vi "PCO_SetCameraSetup.vi"(8 "error in (no error)":errorcluster {"code" format="%x"}, 9 "dwSetup":u32[](array[numeric]), 10 "wType":u16, 11 "ph":u64) -> (0 "error out":errorcluster {"code" format="%x"}, 2 "ErrorMessage":i32 format="%x", 3 "ph out":u64)   [LabVIEW 2019, in "SDK.lvlib" / "GeneralCameraControl.lvlib"]
doc: "<b>Description</b>\nCommand can be used to set the shutter mode of a pco.edge.This function is used to set the operation mode of the camera. If operation mode is changed, PCO_RebootCamera must be called afterwards. It is recommended to set the command timeout to 2000 ms by calling PCO_SetTimeouts before changing the setup.\n\n<b>Supported camera type:</b>\npco.edge\n\n<b>Descriptor dependency:</b>\nNone"
uses:
  GeneralCameraControl.lvlib
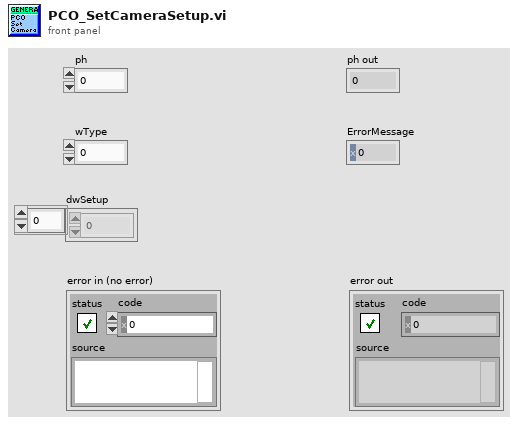
[diagram p1: front panel]
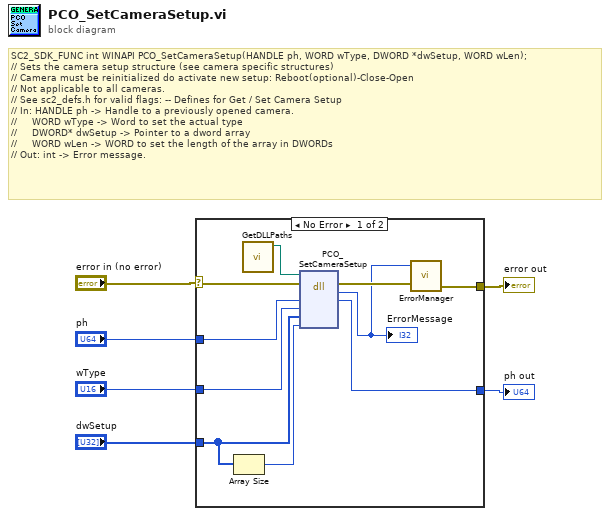
[diagram p0: block diagram]
diagram:
  # "SC2_SDK_FUNC int WINAPI PCO_SetCameraSetup(HANDLE ph, WORD wType, DWORD *dwSetup, WORD wLen);\n// Sets the camera setup structure (see camera specific structures)\n// Camera must be reinitialized do activate new setup: Reboot(optional)-Close-Open\n// Not applicable to all cameras.\n// See sc2_defs.h for valid flags: -- Defines for Get / Set Camera Setup\n// In: HANDLE ph -> Handle to a previously opened camera.\n//     WORD wType -> Word to set the actual type\n//     DWORD* dwSetup -> Pointer to a dword array\n//     WORD wLen -> WORD to set the length of the array in DWORDs\n// Out: int -> Error message."
  n1 = case shown="No Error" "error in (no error)" {
    selector: "error in (no error)" -> [w12 w18]
    tunnel: "ph" -> [w16 w17]
    tunnel: [w15 w17] -> w5
    tunnel: [w14 w18] -> w4
    tunnel: "dwSetup" -> [w9 _]
    tunnel: "wType" -> [w10 _]
    frame No Error {
      n2 = Array Size(array=w9) -> (size(s)=w8:i32)
      n3 = call "GetDLLPaths.vi"() -> ("SC2_Cam_Path"=w7:path)  [unwired: 9 in, 2 out]
      n4 = dll-call lib="?" fn="PCO_SetCameraSetup"(path in=w7, error in=w12, "ph"=w16, "wType"=w10, "dwSetup"=w9, "wLen"=w8) -> (error out=w13:errorcluster, "return type"=w11:i32, "ph"=w15:u64)  [unwired: 4 in, 1 out]
      "ErrorMessage" <- w11
      n5 = call "ErrorManager.vi"("error in (no error)"=w13, "error code"=w11) -> ("error out"=w14:errorcluster)  [unwired: 3 in]
    }
    frame Error {
    }
  }
  "ph out" <- w5
  "error out" <- w4
